vi "Main UI.vi"() -> ()   [LabVIEW 2011]
uses:
  UI typedefs/Progress Bar.ctl
  UI typedefs/Controller Commands.ctl
  UI typedefs/Progress States.ctl
  Procedure Classes/Potting Procedure/Potting Procedure.lvclass
  UI Classes/Console Log/Console Log.lvclass
  UI Classes/Gantry Status/Gantry Status.lvclass
  Shared Components/Gantry Class/Gantry Class.lvclass
panel:
  out "Progress":T1 scale=0.0..8.0
  out "Current Image":T2(plugin-control)
  out "Z Position":dbl(slide) scale=0.0..10.0
  out "XY Position":cluster{dbl, dbl}[](graph)
  in  "Execute Step":bool
  in  "Resume Button":bool
  in  "Suspend Button":bool
  in  "Add Comment":bool
  in  "Comment":string
  in  "Previous Button":bool
  in  "Manual Control":bool
  in  "Emergency Stop":bool
  out "Console":string
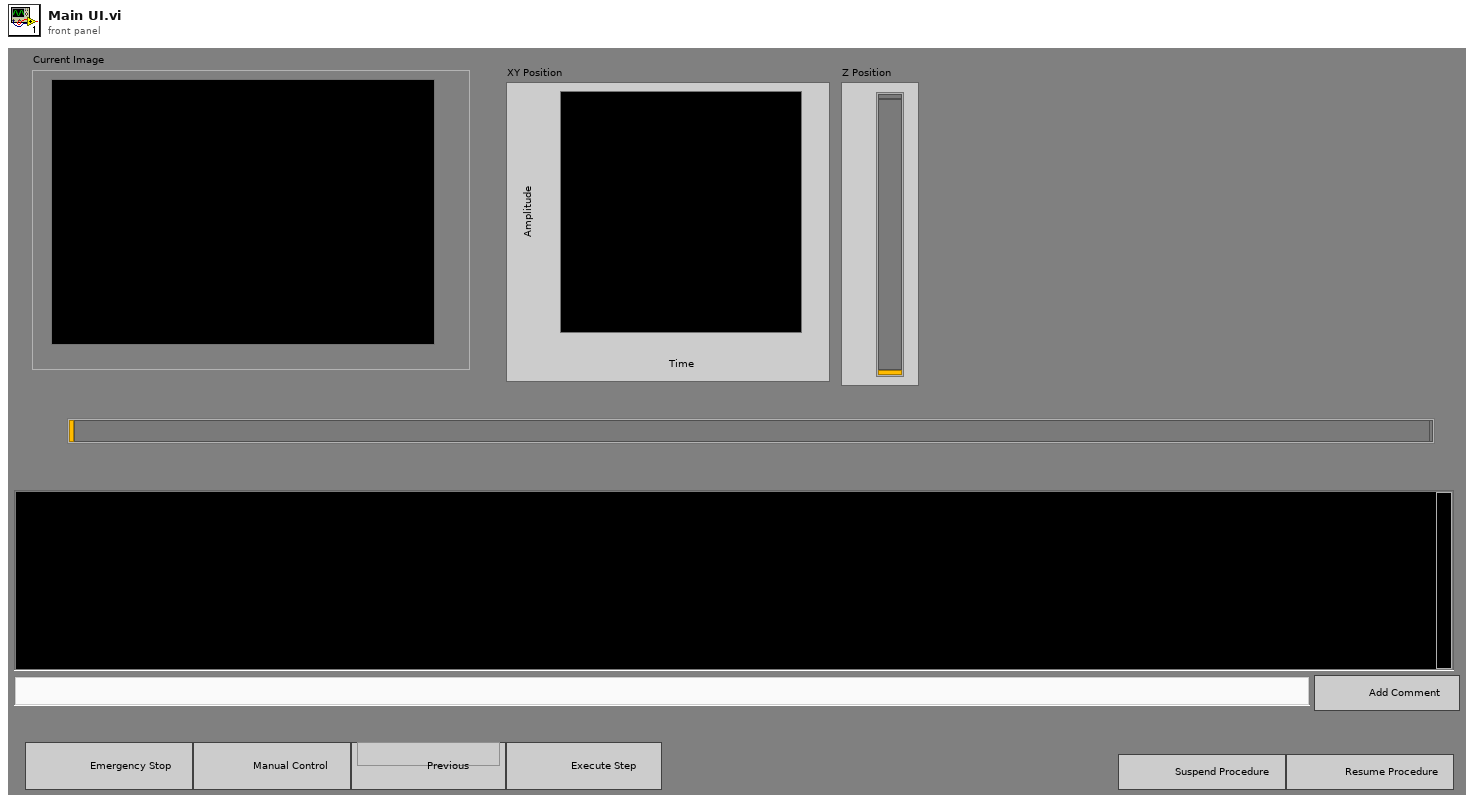
[diagram p1: front panel]
types:
  T1 = typedef "Progress Bar.ctl" = u16
  T2 = typedef "IMAQ Image.ctl" = refnum<image>
  T3 = typedef "Progress States.ctl" = enum16{"Configure Tester", "Inspect Fiducials", "Review Fiducials", "Inspect Modules", "Review Modules", "Fill Sylgard", "Align Needle", "Purge", "Pot"}
  T4 = typedef "Controller Commands.ctl" = enum16{"Initialize", "Execute Step", "Previous Step", "Add Comment", "Manual Control", "Resume", "Pause", "Emergency Stop", "End Procedure"}
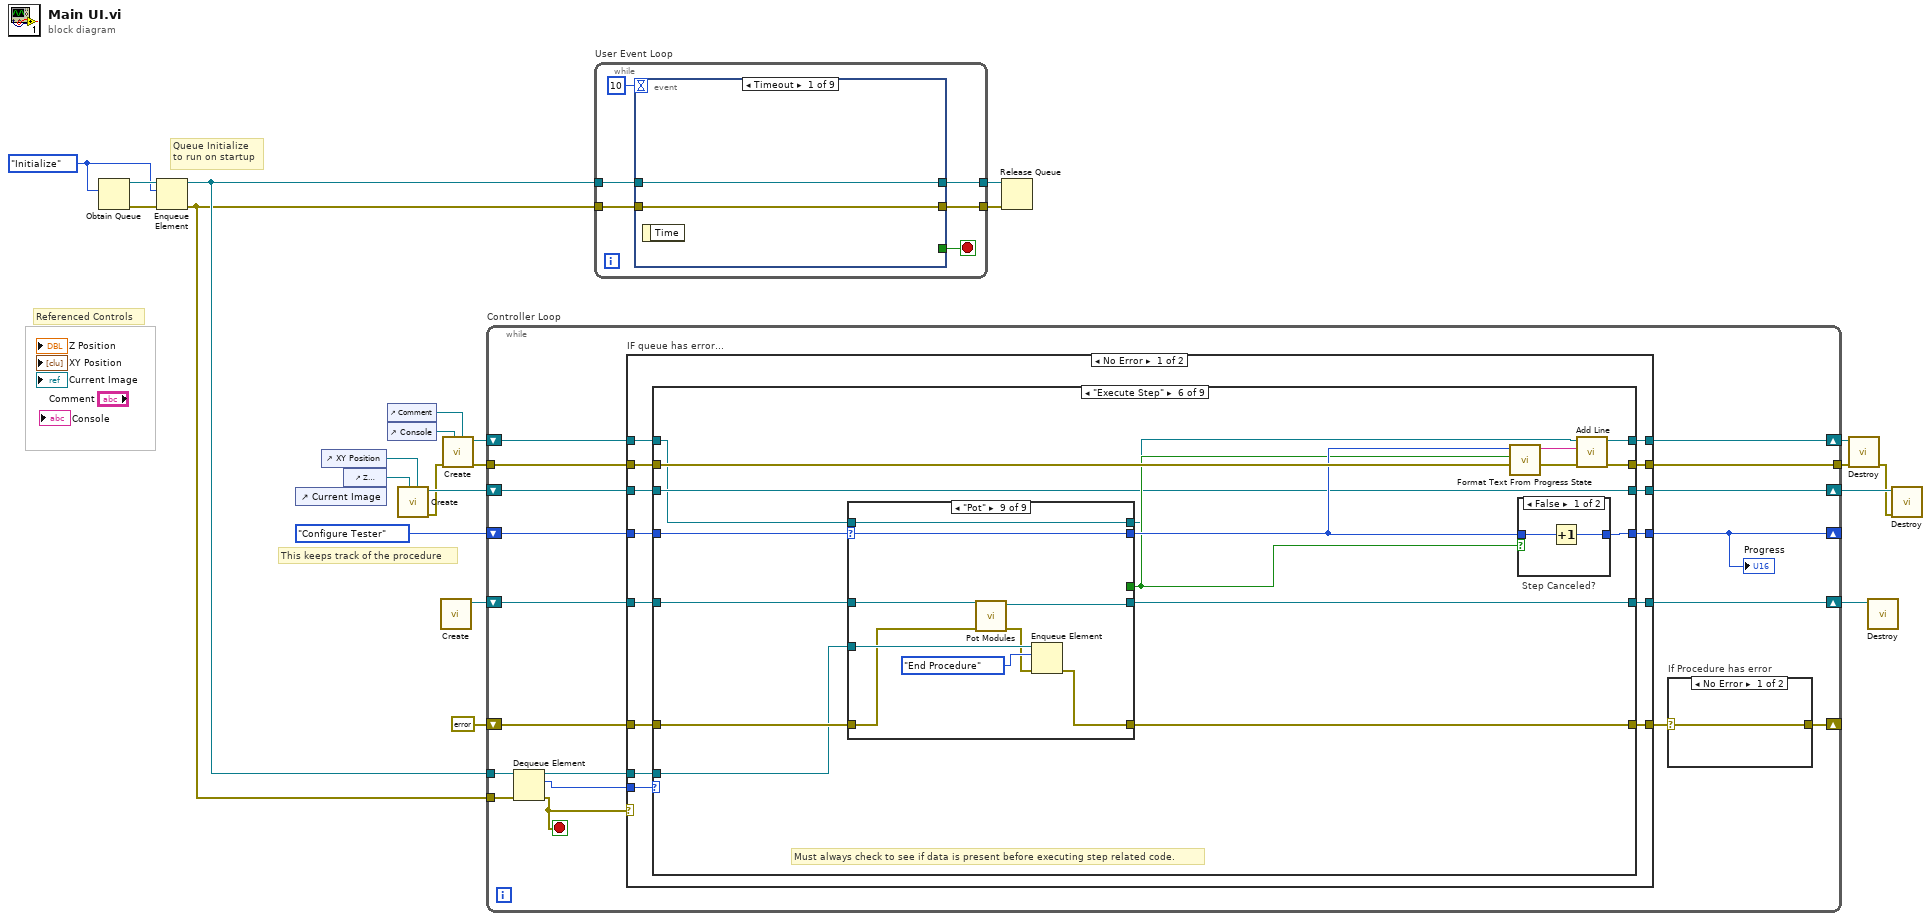
[diagram p0: block diagram]
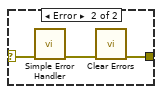
[diagram p2: hidden frame]
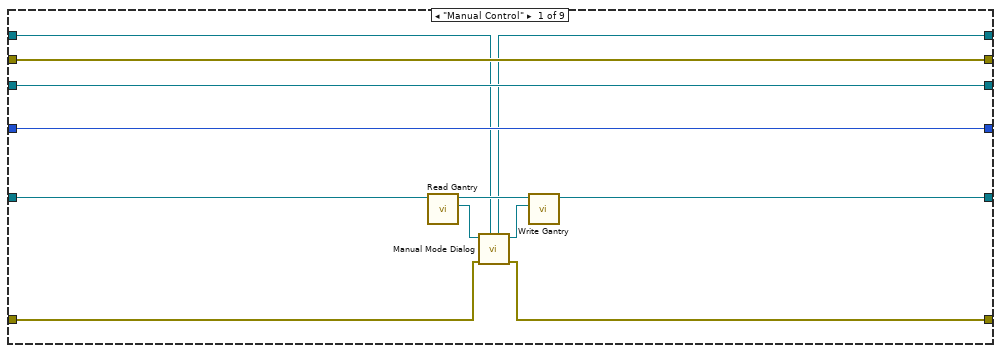
[diagram p3: hidden frame]
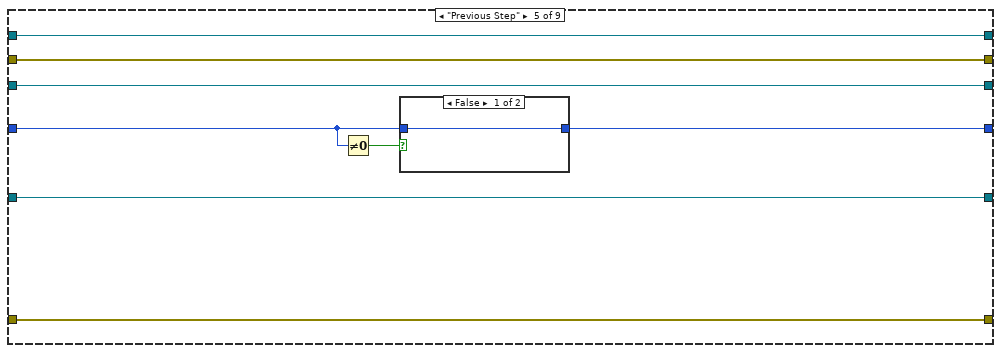
[diagram p7: hidden frame]
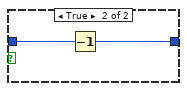
[diagram p8: hidden frame]
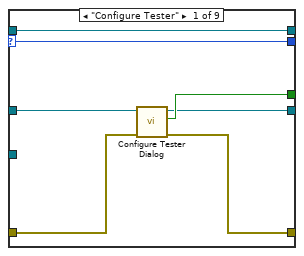
[diagram p10: hidden frame]
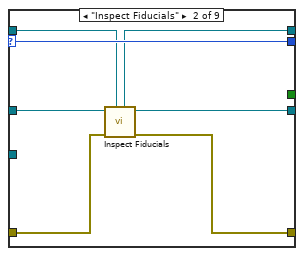
[diagram p11: hidden frame]
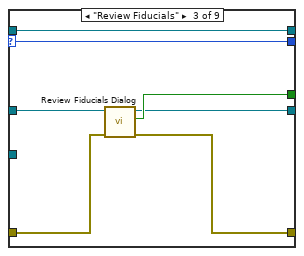
[diagram p12: hidden frame]
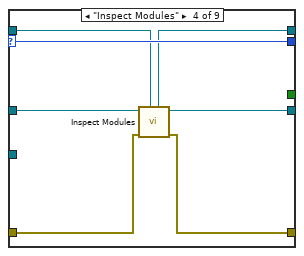
[diagram p13: hidden frame]
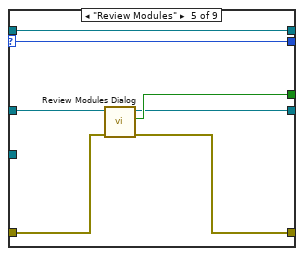
[diagram p14: hidden frame]
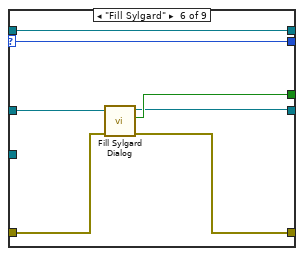
[diagram p15: hidden frame]
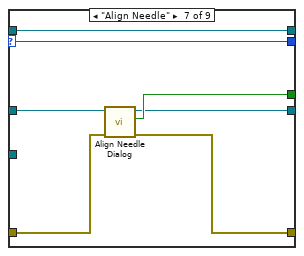
[diagram p16: hidden frame]
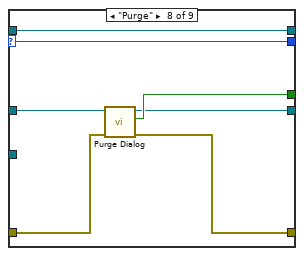
[diagram p17: hidden frame]
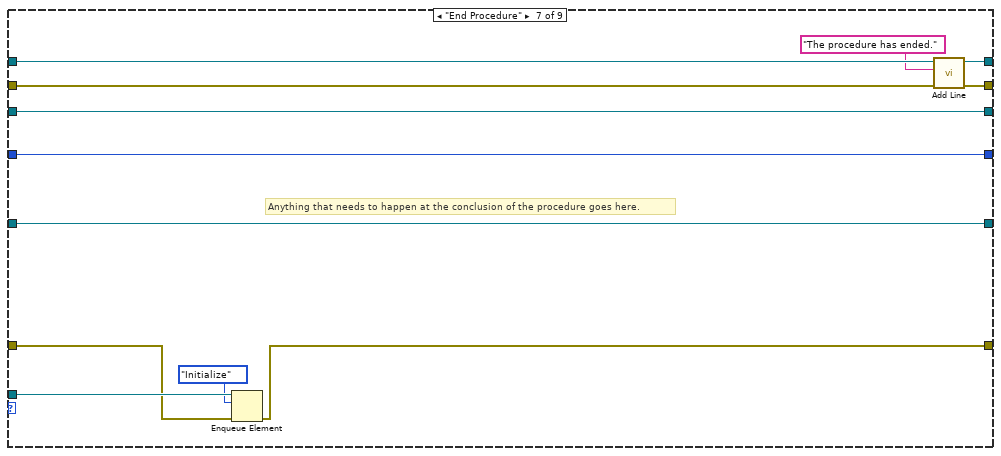
[diagram p18: hidden frame]
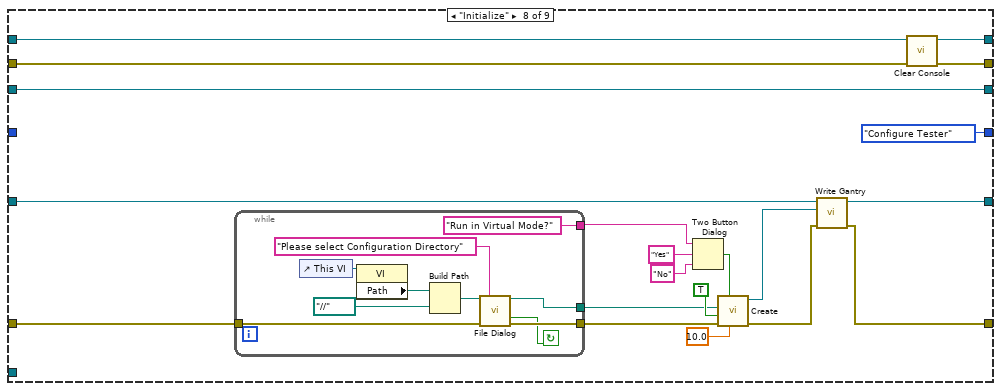
[diagram p19: hidden frame]
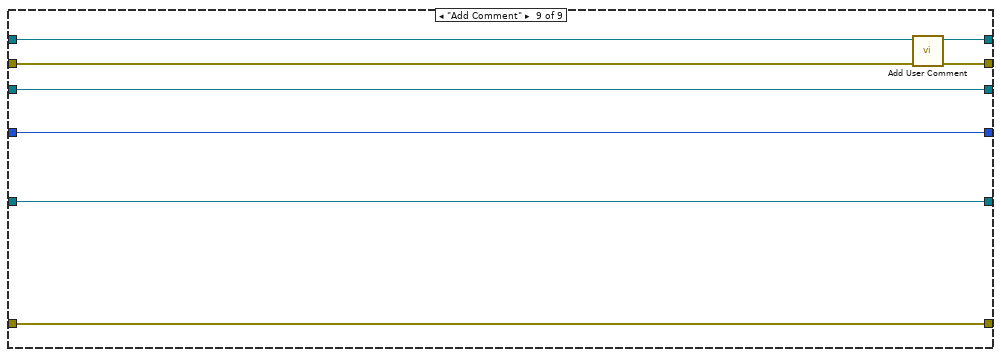
[diagram p20: hidden frame]
diagram:
  w15 = Controller_Commands."Initialize" ("Commands")
  # "Referenced Controls"
  # "This keeps track of the procedure"
  # "Queue Initialize \nto run on startup"
  n1 = Obtain Queue(element data type=w15) -> (queue out=w19:refnum<queue>, error out=w17:errorcluster)  [unwired: 4 in, 1 out]
  n2 = Enqueue Element(queue=w19, element=w15, error in (no error)=w17) -> (queue out=w18:refnum<queue>, error out=w16:errorcluster)  [unwired: 1 in, 1 out]
  n3 = control-ref of="Current Image"() -> ()  [unwired: 1 out]
  n4 = control-ref of="XY Position"() -> (w8:refnum<vi>)
  n5 = control-ref of="Z Position"() -> (w7:refnum<vi>)
  n6 = control-ref of="Comment"() -> (w13:refnum<vi>)
  n7 = control-ref of="Console"() -> (w14:refnum<vi>)
  n8 = call "Create.vi"("XY Position"=w8, "Z Position"=w7) -> ("error out"=w5:errorcluster, "Gantry Status out"=w6:refnum<class "Gantry Status.lvclass">)  [unwired: 8 in]
  n9 = call "Create.vi"() -> ("Potting Procedure out"=w2:refnum<class "Potting Procedure.lvclass">)  [unwired: 10 in, 1 out]
  n10 = call "Create.vi"("Comment"=w13, "Console"=w14, "error in (no error)"=w5) -> ("error out"=w11:errorcluster, "Console Log out"=w12:refnum<class "Console Log.lvclass">)  [unwired: 7 in]
  n11 = while "Controller Loop" {
    tunnel: w16 -> [w41]
    shift-right: [w24] -> _
    shift-left: Progress_States."Configure Tester" -> [w39]
    tunnel: w18 -> [w38]
    shift-right: [w33] -> _
    shift-left: errorcluster {"status"=FALSE, "code"=0, "source"=""} ("error constant") -> [w36]
    tunnel: w11 -> [w30]
    tunnel: [w29] -> w9
    shift-right: [w31] -> w10
    shift-left: w12 -> [w32]
    shift-right: [w27] -> w4
    shift-left: w6 -> [w28]
    shift-right: [w25] -> w1
    shift-left: w2 -> [w26]
    stop <- w35 stop-if-true
    n12 = Dequeue Element(queue=w38, error in (no error)=w41) -> (queue out=w40:refnum<queue>, element=w37:T4, error out=w35:errorcluster)  [unwired: 1 in, 1 out]
    n13 = case "IF queue has error..." shown="No Error" w35 {
      tunnel: w40 -> [w59 _]
      tunnel: w39 -> [w58 w240]
      tunnel: [w57 w240] -> w24
      tunnel: w37 -> [w56 _]
      tunnel: w36 -> [w55 w239]
      tunnel: [w54 w239] -> w34
      tunnel: w32 -> [w53 w238]
      tunnel: [w52 w238] -> w31
      tunnel: w30 -> [w51 w237]
      tunnel: [w50 w237] -> w29
      tunnel: w28 -> [w49 w236]
      tunnel: [w48 w236] -> w27
      tunnel: [w46 w235] -> w25
      tunnel: w26 -> [w47 w235]
      frame No Error {
        n14 = case shown="\"Execute Step\"" w56 {
          tunnel: w59 -> [_ _ _ _ _ w106 w190 _ _]
          tunnel: w58 -> [w71 w77 w83 w89 w91 w116 w196 _ w234]
          tunnel: [w71 w77 w83 w89 w96 w113 w196 Progress_States."Configure Tester" w234] -> w57
          tunnel: w55 -> [w68 w76 w82 w88 w97 w115 w189 w207 w229]
          tunnel: [w67 w76 w82 w88 w97 w114 w188 w202 w229] -> w54
          tunnel: w53 -> [w61 w74 w81 w87 w95 w102 w195 w215 w231]
          tunnel: [w60 w74 w81 w87 w95 w112 w194 w214 w233] -> w52
          tunnel: w51 -> [w70 w75 w80 w86 w94 w111 w193 w213 w230]
          tunnel: [w70 w75 w80 w86 w94 w110 w192 w212 w232] -> w50
          tunnel: w49 -> [w69 w73 w79 w85 w93 w105 w186 w211 w228]
          tunnel: [w69 w73 w79 w85 w93 w105 w186 w211 w228] -> w48
          tunnel: w47 -> [w64 w72 w78 w84 w92 w104 w185 w210 w227]
          tunnel: [w62 w72 w78 w84 w92 w103 w185 w209 w227] -> w46
          frame "Manual Control" {
            n15 = call-dynamic "Read Gantry.vi"("Potting Procedure in"=w64) -> ("Gantry"=w66:refnum<class "Gantry Class.lvclass">, "Potting Procedure out"=w63:refnum<class "Potting Procedure.lvclass">)  [unwired: 8 in, 1 out]
            n16 = call "Manual Mode Dialog.vi"("Console Log in"=w61, "error in"=w68, "Gantry in"=w66) -> ("error out"=w67:errorcluster, "Gantry out"=w65:refnum<class "Gantry Class.lvclass">, "Console Log out"=w60:refnum<class "Console Log.lvclass">)  [unwired: 6 in]
            n17 = call-dynamic "Write Gantry.vi"("Gantry"=w65, "Potting Procedure in"=w63) -> ("Potting Procedure out"=w62:refnum<class "Potting Procedure.lvclass">)  [unwired: 8 in, 1 out]
          }
          frame "Resume" {
            # "Resume will open some sort of file and restore a procedure."
          }
          frame "Pause" {
            # "Pause will cache the state of a procedure to some sort of file."
          }
          frame "Emergency Stop" {
            # "Any actions resultant of an emergency stop goes here."
          }
          frame "Previous Step" {
            n18 = Not Equal To 0?(x=w91) -> (x != 0?=w90:bool)
            n19 = case shown="False" w90 {
              tunnel: w91 -> [w98 w100]
              tunnel: [w98 w99] -> w96
              frame False {
              }
              frame True {
                n20 = Decrement(x=w100) -> (x-1=w99:T3)
              }
            }
          }
          frame "Execute Step" {
            # "Must always check to see if data is present before executing step related code."
            n21 = case shown="\"Pot\"" w116 {
              selector: w116 -> [w124 w133 w140 w147 w154 w161 w168 w175 w184]
              tunnel: [w124 w133 w140 w147 w154 w161 w168 w175 w184] -> w109
              tunnel: w115 -> [w126 w130 w139 w142 w153 w160 w167 w174 w177]
              tunnel: [w125 w129 w138 w141 w152 w159 w166 w173 w181] -> w114
              tunnel: [w123 _ w137 _ w151 w158 w165 w172 _] -> w108
              tunnel: w106 -> [_ _ _ _ _ _ _ _ w183]
              tunnel: w104 -> [w122 w132 w136 w146 w149 w156 w163 w170 w179]
              tunnel: [w121 w131 w135 w145 w148 w155 w162 w169 w178] -> w103
              tunnel: w102 -> [w120 w128 w134 w144 w150 w157 w164 w171 w180]
              tunnel: [w120 w127 w134 w143 w150 w157 w164 w171 w180] -> w101
              frame "Configure Tester" {
                n22 = call "Configure Tester Dialog.vi"("error in"=w126, "Potting Procedure In"=w122) -> ("error out"=w125:errorcluster, "Canceled"=w123:bool, "Potting Procedure Out"=w121:refnum<class "Potting Procedure.lvclass">)  [unwired: 7 in]
              }
              frame "Inspect Fiducials" {
                n23 = call-dynamic "Inspect Fiducials.vi"("Console Log in"=w128, "error in"=w130, "Potting Procedure in"=w132) -> ("error out"=w129:errorcluster, "Potting Procedure out"=w131:refnum<class "Potting Procedure.lvclass">, "Console Log out"=w127:refnum<class "Console Log.lvclass">)  [unwired: 6 in]
              }
              frame "Review Fiducials" {
                n24 = call "Review Fiducials Dialog.vi"("error in"=w139, "Potting Procedure in"=w136) -> ("error out"=w138:errorcluster, "Canceled"=w137:bool, "Potting Procedure out"=w135:refnum<class "Potting Procedure.lvclass">)  [unwired: 7 in]
              }
              frame "Inspect Modules" {
                n25 = call-dynamic "Inspect Modules.vi"("Console Log in"=w144, "error in"=w142, "Potting Procedure in"=w146) -> ("error out"=w141:errorcluster, "Potting Procedure out"=w145:refnum<class "Potting Procedure.lvclass">, "Console Log out"=w143:refnum<class "Console Log.lvclass">)  [unwired: 6 in]
              }
              frame "Review Modules" {
                n26 = call "Review Modules Dialog.vi"("error in"=w153, "Potting Procedure in"=w149) -> ("error out"=w152:errorcluster, "Canceled"=w151:bool, "Potting Procedure out"=w148:refnum<class "Potting Procedure.lvclass">)  [unwired: 7 in]
              }
              frame "Fill Sylgard" {
                n27 = call "Fill Sylgard Dialog.vi"("error in"=w160, "Potting Procedure in"=w156) -> ("error out"=w159:errorcluster, "Canceled"=w158:bool, "Potting Procedure out"=w155:refnum<class "Potting Procedure.lvclass">)  [unwired: 7 in]
              }
              frame "Align Needle" {
                n28 = call "Align Needle Dialog.vi"("error in"=w167, "Potting Procedure in"=w163) -> ("error out"=w166:errorcluster, "Canceled"=w165:bool, "Potting Procedure out"=w162:refnum<class "Potting Procedure.lvclass">)  [unwired: 7 in]
              }
              frame "Purge" {
                n29 = call "Purge Dialog.vi"("error in"=w174, "Potting Procedure in"=w170) -> ("error out"=w173:errorcluster, "Canceled"=w172:bool, "Potting Procedure out"=w169:refnum<class "Potting Procedure.lvclass">)  [unwired: 7 in]
              }
              frame "Pot" {
                n30 = call "Pot Modules.vi"("error in"=w177, "Potting Procedure in"=w179) -> ("error out"=w176:errorcluster, "Potting Procedure out"=w178:refnum<class "Potting Procedure.lvclass">)  [unwired: 8 in]
                n31 = Enqueue Element(queue=w183, element=Controller_Commands."End Procedure", error in (no error)=w176) -> (error out=w181:errorcluster)  [unwired: 1 in, 2 out]
              }
            }
            n32 = call "Format Text From Progress State.vi"("Canceled"=w108, "Enum"=w109) -> ("String"=w107:string)  [unwired: 9 in]
            n33 = case "Step Canceled?" shown="False" w108 {
              tunnel: w109 -> [w118 w119]
              tunnel: [w117 w119] -> w113
              frame False {
                n34 = Increment(x=w118) -> (x+1=w117:T3)
              }
              frame True {
              }
            }
            n35 = call "Add Line.vi"("error in (no error)"=w111, "String"=w107, "Console Log in"=w101) -> ("error out"=w110:errorcluster, "Console Log out"=w112:refnum<class "Console Log.lvclass">)  [unwired: 7 in]
          }
          frame "End Procedure" {
            # "Anything that needs to happen at the conclusion of the procedure goes here."
            n36 = Enqueue Element(queue=w190, element=Controller_Commands."Initialize", error in (no error)=w189) -> (error out=w188:errorcluster)  [unwired: 1 in, 2 out]
            n37 = call "Add Line.vi"("error in (no error)"=w193, "String"="The procedure has ended.", "Console Log in"=w195) -> ("error out"=w192:errorcluster, "Console Log out"=w194:refnum<class "Console Log.lvclass">)  [unwired: 7 in]
          }
          frame "Initialize" {
            n38 = while {
              tunnel: [w225] -> w205
              tunnel: w207 -> [w224]
              tunnel: [w223] -> w204
              tunnel: ["Run in Virtual Mode?" ("T button name (\"OK\")")] -> w198
              stop <- w222 continue-if-true
              n39 = control-ref of="This VI"() -> (w221:refnum<vi>)
              n40 = property class="VI"(reference=w221) -> ("Path"=w220:path)  [unwired: 1 in, 2 out]
              n41 = Build Path(base path=w220, name or relative path=path "../../..") -> (appended path=w218:path)
              n42 = call "File Dialog"("start path"=w218, "prompt"="Please select Configuration Directory", "error in"=w224) -> ("selected path"=w225:path, "cancelled"=w222:bool, "error out"=w223:errorcluster)  [unwired: 9 in, 1 out]
            }
            n43 = Two Button Dialog(message=w198, 1:"No" ("F button name (\"Cancel\")"), 2:"Yes" ("T button name (\"OK\")")) -> (T button?=w201:bool)
            n44 = call "Create.vi"("Speed Limit(mm/s)"=10.0, "Virtual Mode"=w201, "error in"=w204, "HOME?"=TRUE, "Config Folder"=w205) -> ("error out"=w203:errorcluster, "Gantry out"=w208:refnum<class "Gantry Class.lvclass">)  [unwired: 5 in]
            n45 = call-dynamic "Write Gantry.vi"("error in (no error)"=w203, "Gantry"=w208, "Potting Procedure in"=w210) -> ("error out"=w202:errorcluster, "Potting Procedure out"=w209:refnum<class "Potting Procedure.lvclass">)  [unwired: 7 in]
            n46 = call "Clear Console.vi"("error in (no error)"=w213, "Console Log in"=w215) -> ("error out"=w212:errorcluster, "Console Log out"=w214:refnum<class "Console Log.lvclass">)  [unwired: 8 in]
          }
          frame "Add Comment" {
            n47 = call "Add User Comment.vi"("error in (no error)"=w230, "Console Log in"=w231) -> ("error out"=w232:errorcluster, "Console Log out"=w233:refnum<class "Console Log.lvclass">)  [unwired: 8 in]
          }
        }
      }
      frame Error {
      }
    }
    "Progress" <- w24
    n48 = case "If Procedure has error" shown="No Error" w34 {
      selector: w34 -> [w42 w45]
      tunnel: [w42 w44] -> w33
      frame No Error {
      }
      frame Error {
        n49 = call <vilib>:"Simple Error Handler.vi"("error in (no error)"=w45) -> ("error out"=w43:errorcluster)  [unwired: 4 in, 4 out]
        n50 = call <vilib>:"Clear Errors.vi"("error in (no error)"=w43) -> ("error out"=w44:errorcluster)  [unwired: 6 in]
      }
    }
  }
  n51 = while "User Event Loop" {
    tunnel: w18 -> [w241]
    tunnel: [w244] -> w23
    tunnel: w16 -> [w243]
    tunnel: [w242] -> w22
    stop <- w245 stop-if-true
    n52 = event shown="[0] Timeout" {
      selector: _ -> [_ _ _ _ _ _ _ _ _]
      dyn-events: _ -> [_ _ _ _ _ _ _ _ _]
      timeout: 10 -> [_ _ _ _ _ _ _ _ _]
      tunnel: [_ _ _ _ _ _ _ w272 _] -> w245
      tunnel: w241 -> [w248 w250 w254 w260 w262 w267 w269 w271 w278]
      tunnel: [w248 w250 w253 w257 w264 w267 w269 w271 w279] -> w244
      tunnel: w243 -> [w247 w249 w252 w259 w261 w266 w268 w270 w281]
      tunnel: [w247 w249 w251 w258 w263 w266 w268 w270 w280] -> w242
      event Timeout {
        n53 = event-data() -> ()  [unwired: 1 in, 1 out]
      }
      event "Emergency Stop": Mouse Up {
        n54 = event-data() -> ()  [unwired: 1 in, 1 out]
      }
      event "Manual Control": Mouse Up {
        n55 = event-data() -> ()  [unwired: 1 in, 1 out]
        n56 = Enqueue Element(queue=w254, element=Controller_Commands."Manual Control", error in (no error)=w252) -> (queue out=w253:refnum<queue>, error out=w251:errorcluster)  [unwired: 1 in, 1 out]
      }
      event "Execute Step": Mouse Up {
        n57 = event-data() -> ()  [unwired: 1 in, 1 out]
        n58 = Enqueue Element(queue=w260, element=Controller_Commands."Execute Step", error in (no error)=w259) -> (queue out=w257:refnum<queue>, error out=w258:errorcluster)  [unwired: 1 in, 1 out]
      }
      event "Previous Button": Mouse Up {
        n59 = event-data() -> ()  [unwired: 1 in, 1 out]
        n60 = Enqueue Element(queue=w262, element=Controller_Commands."Previous Step", error in (no error)=w261) -> (queue out=w264:refnum<queue>, error out=w263:errorcluster)  [unwired: 1 in, 1 out]
      }
      event "Suspend Button": Mouse Up {
        n61 = event-data() -> ()  [unwired: 1 in, 1 out]
      }
      event "Resume Button": Mouse Up {
        n62 = event-data() -> ()  [unwired: 1 in, 1 out]
      }
      event Panel Close? {
        n63 = event-data() -> ()  [unwired: 1 in, 1 out]
        n64 = Two Button Dialog(message="Are you sure you want to quit?", 1:"Return" ("F button name (\"Cancel\")"), 2:"Quit" ("T button name (\"OK\")")) -> (T button?=w272:bool)
        n65 = event-data("Discard?"=TRUE) -> ()  [unwired: 1 in, 1 out]
      }
      event "Add Comment": Mouse Up {
        n66 = event-data() -> ()  [unwired: 1 in, 1 out]
        n67 = Enqueue Element(queue=w278, element=Controller_Commands."Add Comment", error in (no error)=w281) -> (queue out=w279:refnum<queue>, error out=w280:errorcluster)  [unwired: 1 in, 1 out]
      }
    }
  }
  n68 = Release Queue(queue=w23, error in (no error)=w22) -> ()  [unwired: 1 in, 3 out]
  n69 = call "Destroy.vi"("error in (no error)"=w9, "Console Log in"=w10) -> ("error out"=w3:errorcluster)  [unwired: 8 in, 1 out]
  n70 = call "Destroy.vi"("Potting Procedure in"=w1) -> ()  [unwired: 10 in, 1 out]
  n71 = call "Destroy.vi"("error in (no error)"=w3, "Gantry Status in"=w4) -> ()  [unwired: 9 in, 1 out]
